vi "SIR2.vi"() -> ()   [LabVIEW 2014]
uses:
  <vilib>/Utility/file.llb/Write To Spreadsheet File (DBL).vi
  <vilib>/measure/mamon.llb/Waveform Peak Detection for 1 Chan.vi
  <vilib>/Utility/file.llb/Write To Spreadsheet File (string).vi
  <vilib>/Utility/file.llb/Read From Spreadsheet File (DBL).vi
  <vilib>/measure/NI_MAPro.lvlib
  <vilib>/Utility/file.llb/Read From Spreadsheet File (string).vi
panel:
  out "Feature ampltuides":dbl[][](array[numeric])
  out "Feature positions":dbl[][](array[numeric])
  out "teh data":refnum<data-value>
  out "Wavelengths":dbl[](array[numeric])
  in  "Load data":bool
  out "peaks/valleys":u16(ring) items=["Peaks", "Valleys"]
  out "Zero Ydata":sgl[](array[numeric])
  out "Zero Xdata":sgl[](array[numeric])
  out "ProgBar top":u32(slide) scale=-1.0..3016.0
  out "ProgBar bottom":u8(slide) scale=0.0..100.0
  in  "Run detection":bool
  in  "Delim":string
  out "Files":path[](array[path])
  in  "Ycol":i16=1
  in  "Xcol":i16
  in  "File style":u16(ring) items=["Sequential files", "Single database"]
  in  "Graph tab":T1(tab)
  out "Single scan":cluster{dbl[], dbl[]}[](graph)
  out "File\nname":string
  in  "Save single scan":bool
  in  "File displayed":i32(slide) min=0 max=5 step=1 scale=0.0..5.0
  in  "Save filtered spectras":bool
  out "Intensity Graph":dbl[][](graph)
  in  "Save Intensity plot":bool
  in  "Colour":string(combo)="Hot metal"
  out "Fixed point":cluster{i32[], dbl[]}(graph)
  in  "Save fixed point\ntracking":bool
  in  "Wavelength\nto track":dbl
  out "Closest wavelength":dbl
  out "Wavelength graph":dbl[][](graph)
  in  "Save Features":bool
  out "Intensity graph":dbl[][](graph)
  in  "Feature & tracking tabs":enum32{"Feature detection", "Tracking"}(tab)
  in  "Upper\nThreashold":dbl=20000.0
  in  "Lower\nThreashold":dbl
  in  "Width":dbl=20.0
  in  "2nd Derivative limit":dbl=0.01
  in  "Feature\ntype":string(combo)="1"
  in  "Detection method":string(combo)="0"
  in  "Feature\ndetection":bool
  in  "Open feature settings":bool
  in  "Tracking error limit":dbl=5.0 caption="Tracking error limit (%)"
  in  "Minimum feature length":i32=1
  in  "Tracking":bool
  in  "Tracking\ntype":string(combo)
  in  "Open Button 2":bool
  in  "Crop":bool
  in  "Normalise\nmethod":string(combo)
  in  "Normalise":bool
  in  "Decimate":i32
  in  "Decimate Y/N":bool
  in  "End\nwavelength":sgl
  in  "Start \nwavelength":sgl
  in  "Moving AV":bool
  in  "Transmission":bool
  in  "Load zero":bool
  in  "Moving\naverage":i16=1 min=1 step=1
  out "Number of files":i16
  in  "Load files":bool
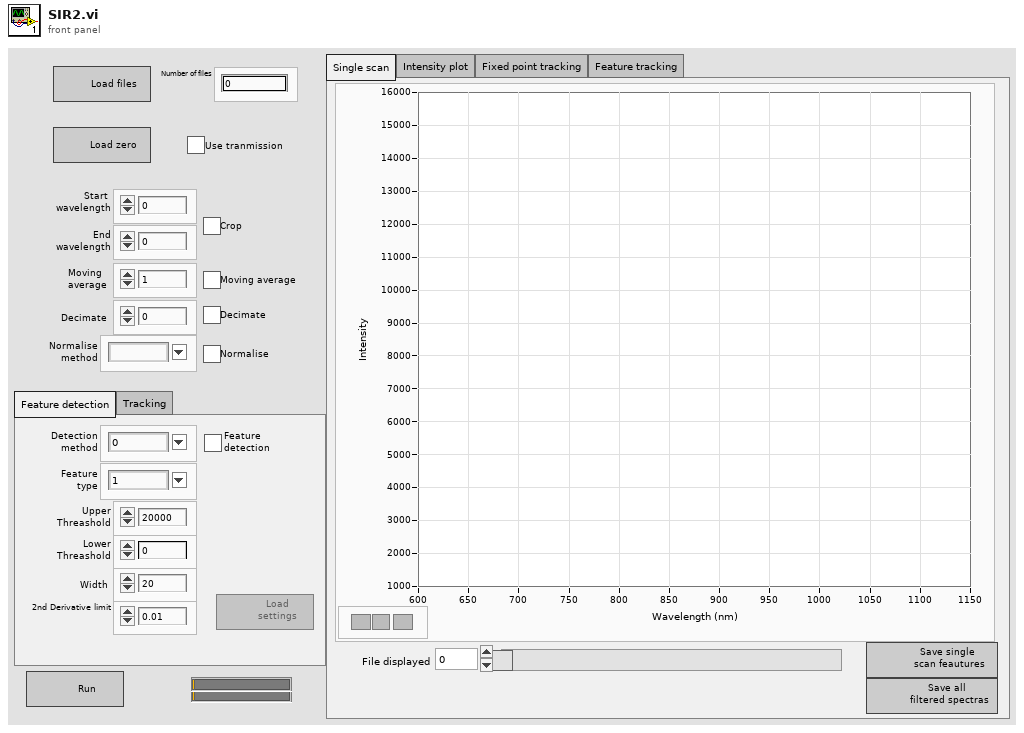
[diagram p1: front panel]
types:
  T1 = enum32{"Single scan", "Intensity plot", "Fixed point tracking", "Feature tracking"}
  T2 = cluster{"Feature positions":dbl[], "Feature ampltuides":dbl[]}
  T3 = cluster{"Feature positions":dbl[], "Feature ampltuides":dbl[]}[]
  T4 = typedef "imagedata.ctl" = cluster{"image type":i32, "image depth":i32, "image":u8[], "mask":u8[], "colors":u32[], "Rectangle":cluster{"left":i16, "top":i16, "right":i16, "bottom":i16}}
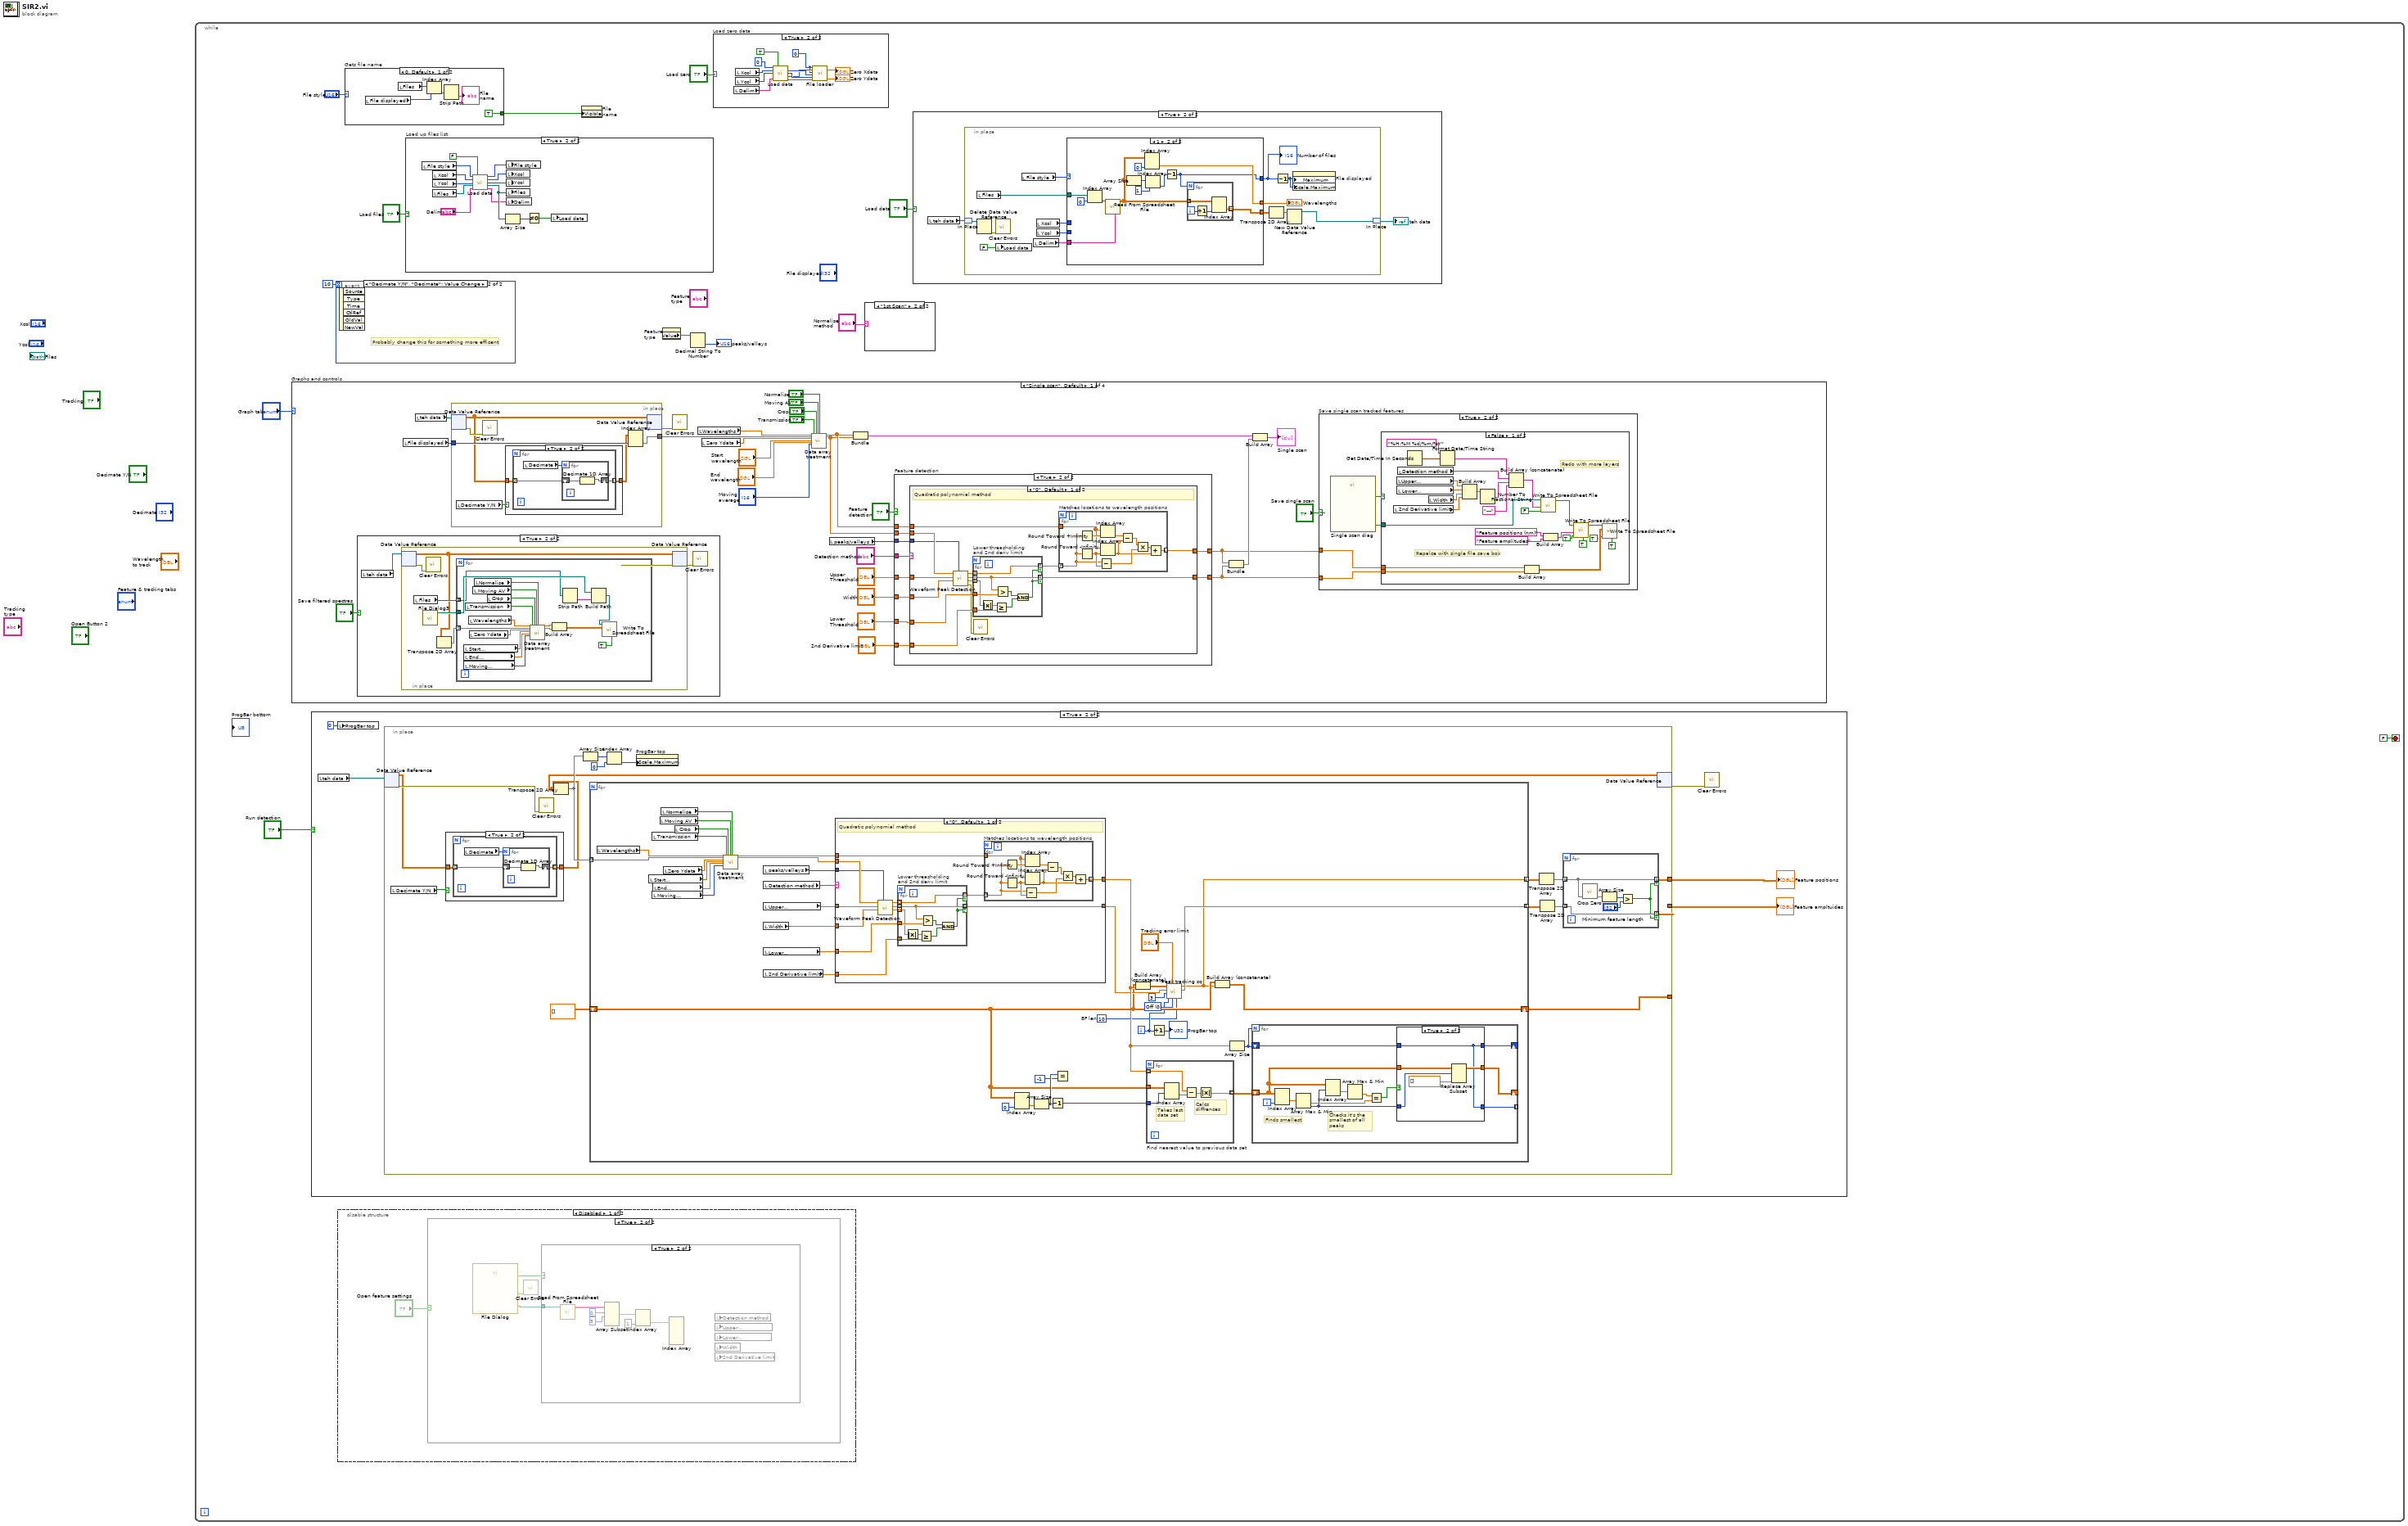
[diagram p0: block diagram]
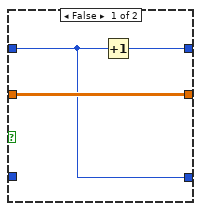
[diagram p7: hidden frame]
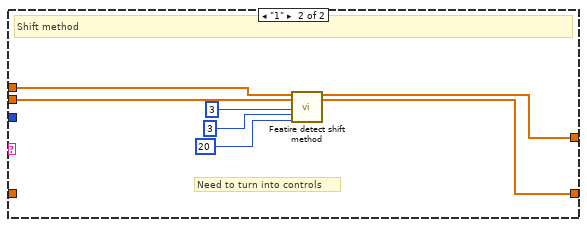
[diagram p8: hidden frame]
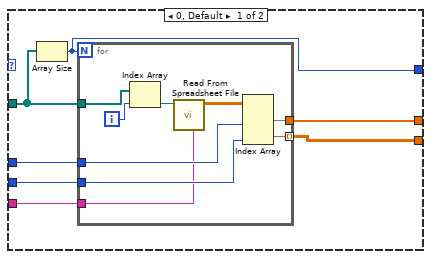
[diagram p10: hidden frame]
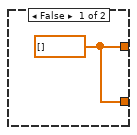
[diagram p17: hidden frame]
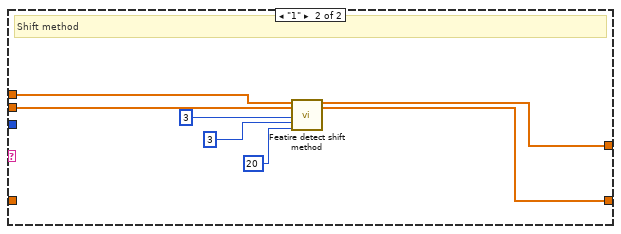
[diagram p18: hidden frame]
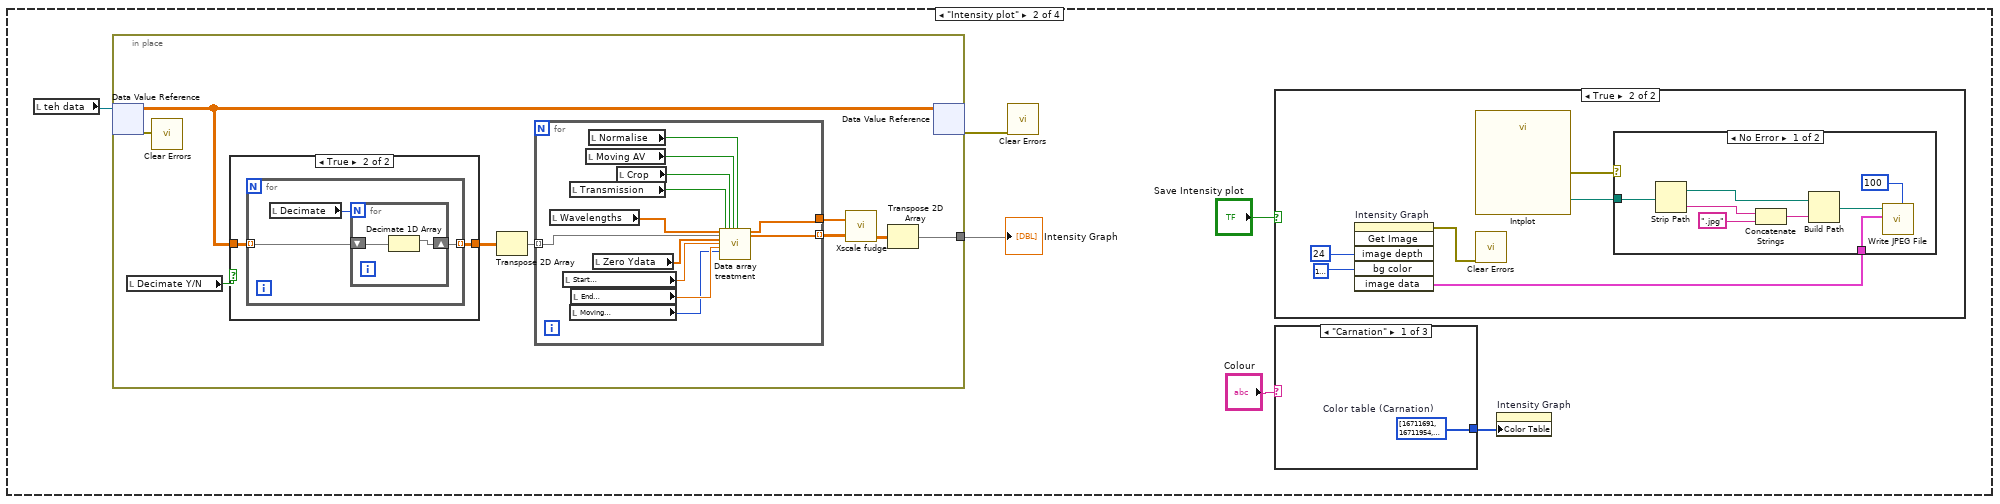
[diagram p19: hidden frame]
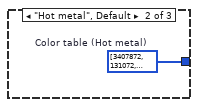
[diagram p20: hidden frame]
diagram:
  n1 = while {
    stop <- FALSE stop-if-true
    n2 = case "Graphs and controls" shown="\"Single scan\", Default" "Graph tab" {
      frame "Single scan", Default {
        n3 = case shown="True" "Save filtered spectras" {
          frame False {
          }
          frame True {
            n4 = local read "teh data"() -> (w252:refnum<data-value>)
            n5 = in-place {
              n6 = in-place-dvr #1(w252) -> (w254:dbl[][], w257:errorcluster)
              n7 = local read "Files"() -> (w256:path[])
              n8 = call "File Dialog3"() -> ("selected path"=w255:path)  [unwired: 12 in, 3 out]
              n9 = call <vilib>:"Clear Errors.vi"("error in (no error)"=w257) -> ()  [unwired: 5 in, 2 out]
              n10 = Transpose 2D Array(2D array=w254) -> (transposed array=w253:dbl[][])
              n11 = for {
                tunnel: w253 -> [w258] mode=indexing
                tunnel: w256 -> [w260] mode=indexing
                tunnel: w255 -> [w261]
                n12 = local read "Start \nwavelength"() -> (w273:sgl)
                n13 = local read "End\nwavelength"() -> (w272:sgl)
                n14 = local read "Moving\naverage"() -> (w271:i16)
                n15 = local read "Transmission"() -> (w270:bool)
                n16 = local read "Wavelengths"() -> (w275:dbl[])
                n17 = local read "Zero Ydata"() -> (w274:sgl[])
                n18 = local read "Moving AV"() -> (w268:bool)
                n19 = local read "Normalise"() -> (w267:bool)
                n20 = local read "Crop"() -> (w269:bool)
                n21 = call "Data array treatment.vi"("Xdata"=w275, "Ydata"=w258, "Zero array"=w274, "Start \nwavelength"=w273, "End\nwavelength"=w272, "Moving\naverage"=w271, "Transmission"=w270, "Crop"=w269, "Moving AV"=w268, "Normalise"=w267) -> ("Xdata"=w266:dbl[], "Ydata"=w265:dbl[])  [unwired: 16 in]
                n22 = Build Array(w266, w265) -> (w264:dbl[][])
                n23 = Strip Path(path=w260) -> (name=w262:string)  [unwired: 1 out]
                n24 = Build Path(base path=w261, name or relative path=w262) -> (appended path=w259:path)
                n25 = call-poly <vilib>:"Write To Spreadsheet File.vi"("transpose? (no:F)"=TRUE, "2D data"=w264, "file path (dialog if empty)"=w259) -> ()  [unwired: 5 in, 1 out]
              }
              n26 = in-place-dvr #1(w254) -> (w251:errorcluster)  [unwired: 1 out]
            }
            n27 = call <vilib>:"Clear Errors.vi"("error in (no error)"=w251) -> ()  [unwired: 5 in, 2 out]
          }
        }
        n28 = local read "File displayed"() -> (w228:i32)
        n29 = local read "teh data"() -> (w230:refnum<data-value>)
        n30 = in-place {
          in-place-border: w228 -> [w309]
          in-place-border: [w310] -> w226
          n31 = in-place-dvr #2(w230) -> (w308:dbl[][], w311:errorcluster)
          n32 = local read "Decimate Y/N"() -> (w306:bool)
          n33 = call <vilib>:"Clear Errors.vi"("error in (no error)"=w311) -> ()  [unwired: 5 in, 2 out]
          n34 = case shown="True" w306 {
            tunnel: w308 -> [w312 w314]
            tunnel: [w312 w313] -> w307
            frame False {
            }
            frame True {
              n35 = for {
                tunnel: [w316] -> w313 mode=indexing
                tunnel: w314 -> [w315] mode=indexing
                n36 = local read "Decimate"() -> (w317:i32)
                n37 = for {
                  N: w317 -> [_]
                  shift-right: [w318] -> w316
                  shift-left: w315 -> [w319]
                  n38 = Decimate 1D Array(w319) -> (w318:dbl[])  [unwired: 1 out]
                }
              }
            }
          }
          n39 = Index Array(array=w307, index (col)=w309) -> (element=w310:dbl[])  [unwired: 1 in]
          n40 = in-place-dvr #2(w308) -> (w229:errorcluster)  [unwired: 1 out]
        }
        n41 = call <vilib>:"Clear Errors.vi"("error in (no error)"=w229) -> ()  [unwired: 5 in, 2 out]
        n42 = local read "Wavelengths"() -> (w227:dbl[])
        n43 = local read "Zero Ydata"() -> (w231:sgl[])
        n44 = call "Data array treatment.vi"("Xdata"=w227, "Ydata"=w226, "Zero array"=w231, "Start \nwavelength"="Start \nwavelength", "End\nwavelength"="End\nwavelength", "Moving\naverage"="Moving\naverage", "Transmission"="Transmission", "Crop"="Crop", "Moving AV"="Moving AV", "Normalise"="Normalise") -> ("Xdata"=w240:dbl[], "Ydata"=w239:dbl[])  [unwired: 16 in]
        n45 = local read "peaks/valleys"() -> (w248:u16)
        n46 = Bundle("Xdata"=w240, "Ydata"=w239) -> (w241:cluster{"Xdata":dbl[], "Ydata":dbl[]})  [unwired: 1 in]
        n47 = case "Feature detection" shown="True" "Feature\ndetection" {
          tunnel: w240 -> [_ w329]
          tunnel: w239 -> [_ w328]
          tunnel: "Detection method" -> [_ w330]
          tunnel: w248 -> [_ w327]
          tunnel: "Upper\nThreashold" -> [_ w326]
          tunnel: "Width" -> [_ w325]
          tunnel: "Lower\nThreashold" -> [_ w324]
          tunnel: "2nd Derivative limit" -> [_ w323]
          tunnel: [w320 w322] -> w224
          tunnel: [w320 w321] -> w223
          frame False {
            w320 = dbl[] []
          }
          frame True {
            n48 = case shown="\"0\", Default" w330 {
              tunnel: w329 -> [w334 w370]
              tunnel: w328 -> [w344 w369]
              tunnel: w327 -> [w343 _]
              tunnel: w326 -> [w342 _]
              tunnel: w325 -> [w341 _]
              tunnel: w324 -> [w337 _]
              tunnel: w323 -> [w336 _]
              tunnel: [w333 w368] -> w321
              tunnel: [w332 w367] -> w322
              frame "0", Default {
                # "Quadratic polynomial method"
                n49 = call-poly <vilib>:"Waveform Peak Detection.vi"("peaks/valleys"=w343, "width"=w341, "threshold"=w342, "Signal In"=w344) -> ("error out"=w331:errorcluster, "2nd Derivatives"=w338:dbl[], "Amplitudes"=w339:dbl[], "Locations"=w340:dbl[])  [unwired: 3 in, 1 out]
                n50 = for "Lower threasholding\nand 2nd deriv limit" {
                  tunnel: w340 -> [w362] mode=indexing
                  tunnel: w339 -> [w361] mode=indexing
                  tunnel: w338 -> [w355] mode=indexing
                  tunnel: w337 -> [w363]
                  tunnel: [w362] -> w335 mode=indexing if=w360
                  tunnel: [w361] -> w332 mode=indexing if=w360
                  tunnel: w336 -> [w359]
                  n51 = Absolute Value(x=w355) -> (abs(x)=w356:dbl)
                  n52 = Greater Or Equal?(x=w356, y=w359) -> (x >= y?=w358:bool)
                  n53 = Greater?(x=w361, y=w363) -> (0:w357:bool)
                  n54 = And(x=w357, y=w358) -> (x .and. y?=w360:bool)
                }
                n55 = call <vilib>:"Clear Errors.vi"("error in (no error)"=w331) -> ()  [unwired: 5 in, 2 out]
                n56 = for "Matches locations to wavelength positions" {
                  tunnel: w335 -> [w346] mode=indexing
                  tunnel: w334 -> [w347]
                  tunnel: [w345] -> w333 mode=indexing
                  n57 = Round Toward +Infinity ("Round To +Infinity")(x=w346) -> (ceil(x): smallest int >= x=w354:dbl)
                  n58 = Round Toward -Infinity ("Round To -Infinity")(1:w346) -> (0:w353:dbl)
                  n59 = Subtract(x=w346, y=w353) -> (x-y=w350:dbl)
                  n60 = Index Array(array=w347, index=w354) -> (element=w352:dbl)
                  n61 = Index Array(array=w347, index=w353) -> (element=w348:dbl)
                  n62 = Subtract(x=w352, y=w348) -> (x-y=w351:dbl)
                  n63 = Multiply(x=w351, y=w350) -> (x*y=w349:dbl)
                  n64 = Add(x=w349, y=w348) -> (x+y=w345:dbl)
                }
              }
              frame "1" {
                # "Shift method"
                n65 = call "Featire detect shift method.vi"("Xvalues"=w370, "Yvalues"=w369, "magnitude  limit"=3, "Shift"=3, "Window"=20) -> ("Feature positions"=w368:dbl[], "Feature ampltuides"=w367:dbl[])  [unwired: 13 in]
              }
            }
          }
        }
        n66 = Bundle("Feature positions"=w223, "Feature ampltuides"=w224) -> (w242:T2)  [unwired: 1 in]
        n67 = Build Array(w241, w242) -> (→"Single scan":T3)
        n68 = case "Save single scan tracked features" shown="True" "Save single scan" {
          tunnel: w224 -> [_ w277]
          tunnel: w223 -> [_ w276]
          frame False {
          }
          frame True {
            n69 = call "Single scan diag"() -> ("selected path"=w279:path, "cancelled"=w278:bool)  [unwired: 12 in, 2 out]
            n70 = case shown="False" w278 {
              tunnel: w279 -> [w287 _]
              tunnel: w277 -> [w296 _]
              tunnel: w276 -> [w295 _]
              frame False {
                # "Repalce with single file save box"
                # "Redo with more layers"
                n71 = local read "2nd Derivative limit"() -> (w291:dbl)
                n72 = local read "Upper\nThreashold"() -> (w288:dbl)
                n73 = local read "Lower\nThreashold"() -> (w289:dbl)
                n74 = local read "Detection method"() -> (w293:string)
                n75 = Get Date/Time In Seconds() -> (seconds since 1Jan1904=w282:timestamp)
                n76 = local read "Width"() -> (w290:dbl)
                n77 = Format Date/Time String(time format string (%c)="%H:%M %d/%m/%Y", seconds (now)=w282) -> (date/time string=w283:string)  [unwired: 1 in]
                n78 = Build Array(w288, w289, w290, w291) -> (w292:dbl[])
                n79 = Number To Fractional String(number=w292) -> (F-format string=w294:string[])  [unwired: 3 in]
                n80 = Build Array (concatenate)(w283, w293, w294, "---") -> (w285:string[])
                n81 = Build Array(w295, w296) -> (w300:dbl[][])
                n82 = call-poly <vilib>:"Write To Spreadsheet File.vi"("append to file? (new file:F)"=FALSE, "1D data"=w285, "file path (dialog if empty)"=w287) -> ("new file path (Not A Path if cancelled)"=w286:path)  [unwired: 5 in]
                n83 = Build Array("Feature positions (nm)", "Feature amplitudes") -> (w299:string[])
                n84 = call-poly <vilib>:"Write To Spreadsheet File.vi"("transpose? (no:F)"=TRUE, "append to file? (new file:F)"=TRUE, "1D data"=w299, "file path (dialog if empty)"=w286) -> ("new file path (Not A Path if cancelled)"=w305:path)  [unwired: 4 in]
                n85 = call-poly <vilib>:"Write To Spreadsheet File.vi"("transpose? (no:F)"=TRUE, "append to file? (new file:F)"=TRUE, "2D data"=w300, "file path (dialog if empty)"=w305) -> ()  [unwired: 4 in, 1 out]
              }
              frame True {
              }
            }
          }
        }
      }
      frame "Intensity plot" {
        n86 = local read "teh data"() -> (w376:refnum<data-value>)
        n87 = in-place {
          in-place-border: [w399] -> w374
          n88 = in-place-dvr #3(w376) -> (w394:dbl[][], w398:errorcluster)
          n89 = local read "Decimate Y/N"() -> (w396:bool)
          n90 = call <vilib>:"Clear Errors.vi"("error in (no error)"=w398) -> ()  [unwired: 5 in, 2 out]
          n91 = case shown="True" w396 {
            tunnel: [w403 w405] -> w395
            tunnel: w394 -> [w403 w404]
            frame False {
            }
            frame True {
              n92 = for {
                tunnel: [w407] -> w405 mode=indexing
                tunnel: w404 -> [w406] mode=indexing
                n93 = local read "Decimate"() -> (w408:i32)
                n94 = for {
                  N: w408 -> [_]
                  shift-right: [w409] -> w407
                  shift-left: w406 -> [w410]
                  n95 = Decimate 1D Array(w410) -> (w409:dbl[])  [unwired: 1 out]
                }
              }
            }
          }
          n96 = Transpose 2D Array(2D array=w395) -> (transposed array=w397:dbl[][])
          n97 = for {
            tunnel: [w414] -> w402 mode=indexing
            tunnel: [w413] -> w401
            tunnel: w397 -> [w412] mode=indexing
            n98 = local read "Wavelengths"() -> (w411:dbl[])
            n99 = local read "Start \nwavelength"() -> (w418:sgl)
            n100 = local read "Transmission"() -> (w419:bool)
            n101 = local read "Moving\naverage"() -> (w416:i16)
            n102 = local read "End\nwavelength"() -> (w417:sgl)
            n103 = local read "Moving AV"() -> (w421:bool)
            n104 = local read "Normalise"() -> (w422:bool)
            n105 = local read "Zero Ydata"() -> (w415:sgl[])
            n106 = local read "Crop"() -> (w420:bool)
            n107 = call "Data array treatment.vi"("Xdata"=w411, "Ydata"=w412, "Zero array"=w415, "Start \nwavelength"=w418, "End\nwavelength"=w417, "Moving\naverage"=w416, "Transmission"=w419, "Crop"=w420, "Moving AV"=w421, "Normalise"=w422) -> ("Xdata"=w413:dbl[], "Ydata"=w414:dbl[])  [unwired: 16 in]
          }
          n108 = call "Xscale fudge.vi"("x array"=w401, "intensity array in"=w402) -> ("intensity array out"=w400:dbl[][])  [unwired: 2 out]
          n109 = Transpose 2D Array(2D array=w400) -> (transposed array=w399:dbl[][])
          n110 = in-place-dvr #3(w394) -> (w375:errorcluster)  [unwired: 1 out]
        }
        "Intensity Graph" <- w374
        n111 = call <vilib>:"Clear Errors.vi"("error in (no error)"=w375) -> ()  [unwired: 5 in, 2 out]
        n112 = case shown="True" "Save Intensity plot" {
          frame False {
          }
          frame True {
            n113 = invoke on="Intensity Graph" class="IntGraph (strict)" method="Get Image"("image depth"=24 ("Image Depth"), "bg color"=u32 16777225) -> (error out=w383:errorcluster, "image data"=w382:T4)  [unwired: 4 in, 4 out]
            n114 = call "Intplot"() -> ("selected path"=w381:path, "error out"=w384:errorcluster)  [unwired: 12 in, 2 out]
            n115 = call <vilib>:"Clear Errors.vi"("error in (no error)"=w383) -> ()  [unwired: 5 in, 2 out]
            n116 = case shown="No Error" w384 {
              tunnel: w381 -> [w392 _]
              tunnel: w382 -> [w386 _]
              frame No Error {
                n117 = Strip Path(path=w392) -> (stripped path=w388:path, name=w390:string)
                n118 = Concatenate Strings(w390, ".jpg") -> (w389:string)
                n119 = Build Path(base path=w388, name or relative path=w389) -> (appended path=w387:path)
                n120 = call <vilib>:"Write JPEG File.vi"("quality (80)"=100, "image data"=w386, "path to JPEG file"=w387) -> ()  [unwired: 7 in, 2 out]
              }
              frame Error {
              }
            }
          }
        }
        n121 = case shown="\"Carnation\"" "Colour" {
          tunnel: [w377 w378 w379] -> w371
          frame "Carnation" {
            w377 = u32[] [16711691, 16711954, 16712217, 16712480, 16712742, 16713005, 16713268, 16713530, 16713793, 16714056, 16715086, 16714580, 16714842, 16715104, 16715367, 16715629, 16715891, 16716153, 16716415, 16716677, 16716940, 16717202, 16717463, 16717725, 16717987, 16718249, 16718511, 16718772, 16719034, 16719296, 16719557, 16719819, 16720079, 16720341, 16720602, 16720863, 16721125, 16721386, 16721647, 16721908, 16722169, 16722430, 16395007, 16133119, 15805695, 15478271, 15216383, 14888959, 14561535, 14234111, 13972223, 13644799, 13382911, 13055487, 12793599, 12531711, 12269823, 11942399, 11680511, 11418623, 11156735, 10829311, 10567423, 10305535, 10305535, 10043647, 9781503, 9585151, 9323263, 9061375, 8799487, 8537599, 8341247, 8079359, 7883007, 7621119, 7424767, 7228415, 6966527, 6770175, 6573823, 6377471, 6115583, 5919231, 5722879, 5526527, 5527551, 5594111, 5660927, 5727743, 5794559, 5861375, 5927935, 5994751, 6061567, 6128127, 6194943, 6261503, 6328063, 6394879, 6461439, 6527999, 6594815, 6661375, 6727935, 6794495, 6861055, 6927871, 6994175, 7060735, 7127295, 7193855, 7260415, 7326719, 7393279, 7459839, 7526143, 7592703, 7659007, 7725311, 7791871, 7858175, 7924479, 7991039, 8057343, 8123647, 8189951, 8256255, 8322815, 8388605, 8454139, 8519672, 8585205, 8650738, 8716271, 8781804, 8847338, 8912871, 8978404, 9043938, 9109472, 9175005, 9240539, 9306073, 9371606, 9437140, 9502674, 9568208, 9633742, 9699275, 9764809, 9830343, 9895877, 9961412, 10026946, 10092480, 10158014, 10223548, 10289083, 10354617, 10420152, 10485686, 10551221, 10616755, 10682290, 10747825, 10813359, 10878894, 10944429, 11009964, 11075499, 11141034, 11206570, 11403179, 11599788, 11796397, 11993006, 12124079, 12320688, 12517297, 12648370, 12844979, 13041588, 13172661, 13303734, 13500343, 13631416, 13762489, 13959098, 14090171, 14221244, 14352317, 14352317, 14483390, 14614463, 14745535, 14876608, 15007681, 15138754, 15269827, 15335364, 15466437, 15597510, 15663047, 15794120, 15859657, 15990730, 16056267, 16121804, 16252877, 16318414, 16383951, 16515024, 16580561, 16646098, 16711635, 16776916, 16776917, 16776662, 16776407, 16776152, 16775897, 16775642, 16775643, 16775388, 16775133, 16775134, 16775135, 16774880, 16774881, 16774626, 16774627, 16774628, 16774373, 16774374, 16774375, 16774376, 16774377, 16774378, 16774379, 16774380, 16774381, 16774638, 16774639, 16774640, 16774641, 16774898, 16774899, 16775156, 16775157, 16775414, 16775415, 16775672, 16775929, 16776186, 16776187]  # Color table (Carnation)
          }
          frame "Hot metal", Default {
            w378 = u32[] [3407872, 131072, 196608, 327680, 458752, 589824, 655360, 786432, 917504, 1048576, 1114112, 1245184, 1376256, 1507328, 1572864, 1703936, 1835008, 1966080, 2031616, 2162688, 2293760, 2424832, 2555904, 2621440, 2752512, 2883584, 3014656, 3080192, 3211264, 3342336, 3473408, 3538944, 3670016, 3801088, 3932160, 3997696, 4128768, 4259840, 4390912, 4456448, 4587520, 4718592, 4849664, 4980736, 5046272, 5177344, 5308416, 5439488, 5505024, 5636096, 5767168, 5898240, 5963776, 6094848, 6225920, 6356992, 6422528, 6553600, 6684672, 6815744, 6881280, 7012352, 7143424, 7143424, 7274496, 7405568, 7471104, 7602176, 7733248, 7864320, 7929856, 8060928, 8192000, 8323072, 8388608, 8519680, 8650752, 8781824, 8847360, 8978432, 9109504, 9240576, 9306112, 9437184, 9568256, 9699328, 9830400, 9895936, 10027008, 10158080, 10289152, 10354688, 10485760, 10616832, 10747904, 10813440, 10944512, 11075584, 11206656, 11272192, 11403264, 11534336, 11665408, 11730944, 11862016, 11993088, 12124160, 12189696, 12320768, 12451840, 12582912, 12713984, 12779520, 12910592, 13041664, 13172736, 13238272, 13369344, 13500416, 13631488, 13697024, 13828096, 13959168, 14090240, 14155776, 14286848, 14417920, 14548992, 14614528, 14745600, 14876672, 15007744, 15138816, 15204352, 15335424, 15466496, 15597568, 15663104, 15794176, 15925248, 16056320, 16121856, 16252928, 16384000, 16515072, 16580608, 16580608, 16580608, 16515072, 16711680, 16711680, 16711680, 16712192, 16647424, 16713728, 16714496, 16715264, 16716032, 16716800, 16717568, 16718336, 16719104, 16719872, 16720640, 16721408, 16722176, 16722944, 16723712, 16724480, 16725248, 16726016, 16726784, 16727552, 16728064, 16728832, 16729600, 16730368, 16731136, 16731904, 16732672, 16733440, 16734208, 16734976, 16735744, 16736512, 16737280, 16738048, 16738816, 16739584, 16740352, 16741120, 16741120, 16741888, 16742656, 16743424, 16743936, 16744704, 16745472, 16746240, 16747008, 16747776, 16748544, 16749312, 16750080, 16750848, 16751616, 16752384, 16753152, 16753920, 16754688, 16755456, 16756224, 16756992, 16757760, 16758528, 16759296, 16760064, 16760576, 16761344, 16762112, 16762880, 16763648, 16764416, 16765184, 16765952, 16766720, 16767488, 16768256, 16769024, 16769792, 16770560, 16771328, 16772096, 16772864, 16773632, 16774400, 16775168, 16775936, 16776448, 16776960, 16776960, 16776960, 16776960, 16776960, 16776960, 16776960, 16776960, 16776960, 16776960, 16776960, 16776960, 16776960, 16776960, 16776960, 16776448]  # Color table (Hot metal)
          }
          frame "Rainbow-striped" {
            w379 = u32[] [12255418, 12386492, 12517567, 12320960, 12189888, 12058817, 11927746, 11731139, 11600067, 9175197, 9044125, 11141318, 11010246, 10813639, 10682568, 10551497, 10354890, 10223818, 10092747, 7930019, 7798948, 9633997, 9502926, 9306319, 9175248, 9044176, 8847569, 8716498, 8585427, 6750377, 6619306, 8126677, 7995606, 7798999, 7667927, 7536856, 7340249, 7209178, 7078106, 5505199, 5374128, 6619357, 6488285, 6291678, 6160607, 6029536, 5832929, 5701857, 5570786, 4325557, 4194486, 5112036, 4980965, 4784358, 4653287, 4522215, 4325608, 4194537, 4063466, 3080380, 3014844, 3604716, 3408109, 3277038, 3277038, 3145966, 3014895, 2818288, 2687217, 2556145, 1900738, 1769666, 2097396, 1900789, 1769717, 1638646, 1507575, 1310968, 1179896, 1048825, 721096, 590024, 590075, 393468, 262397, 131326, 255, 1791, 3327, 4863, 5068, 6348, 9471, 11007, 12543, 14079, 15615, 17151, 18687, 20223, 17612, 18636, 25087, 26623, 28159, 29695, 31231, 32767, 34303, 35839, 29900, 31180, 40447, 41983, 43775, 45311, 46847, 48383, 49919, 51455, 42444, 43724, 56063, 57599, 59135, 60671, 62207, 63743, 65535, 65528, 52418, 52413, 65510, 65504, 65498, 65492, 65486, 65480, 65474, 65468, 52369, 52364, 65449, 65443, 65437, 65431, 65425, 65419, 65413, 65407, 52321, 52316, 65389, 65383, 65377, 65371, 65364, 65358, 65352, 65346, 52272, 52267, 65328, 65322, 65316, 65310, 65304, 65298, 65292, 65286, 52224, 314368, 851712, 1244928, 1638144, 2031360, 2424576, 2817792, 3211008, 3604224, 3197952, 3525632, 4783872, 5177088, 5635840, 6029056, 6422272, 6815488, 7208704, 7601920, 6409216, 6736896, 6736896, 8781568, 9174784, 9568000, 9961216, 10354432, 10747648, 11206400, 11599616, 9554944, 9882624, 12779264, 13172480, 13565696, 13958912, 14352128, 14745344, 15138560, 15531776, 12766208, 13093888, 16776960, 16775170, 16773637, 16771847, 16770314, 16768780, 16766991, 16765457, 13411088, 13409810, 16760601, 16758812, 16757278, 16755745, 16753955, 16752422, 16750888, 16749099, 13398052, 13396774, 16744243, 16742704, 16741166, 16739884, 16738345, 16736807, 16735269, 16733730, 13385753, 13384728, 16729371, 16727833, 16726295, 16725012, 16723474, 16721936, 16720397, 16718859, 13373959, 13372677, 16714500, 16712962, 16711680]  # Color table (Rainbow-striped)
          }
        }
        n122 = property on="Intensity Graph" class="IntGraph (strict)"("Color Table"=w371) -> ()  [unwired: 2 in, 2 out]
      }
      frame "Fixed point tracking" {
        n123 = local read "teh data"() -> (w427:refnum<data-value>)
        n124 = in-place {
          in-place-border: [w453] -> w428
          in-place-border: [w446] -> w425
          in-place-border: [w445] -> w423
          n125 = in-place-dvr #4(w427) -> (w448:dbl[][], w451:errorcluster)
          n126 = local read "Decimate Y/N"() -> (w447:bool)
          n127 = call <vilib>:"Clear Errors.vi"("error in (no error)"=w451) -> ()  [unwired: 5 in, 2 out]
          n128 = case shown="True" w447 {
            tunnel: [w455 w457] -> w449
            tunnel: w448 -> [w455 w456]
            frame False {
            }
            frame True {
              n129 = for {
                tunnel: [w459] -> w457 mode=indexing
                tunnel: w456 -> [w458] mode=indexing
                n130 = local read "Decimate"() -> (w460:i32)
                n131 = for {
                  N: w460 -> [_]
                  shift-right: [w461] -> w459
                  shift-left: w458 -> [w462]
                  n132 = Decimate 1D Array(w462) -> (w461:dbl[])  [unwired: 1 out]
                }
              }
            }
          }
          n133 = local read "Wavelengths"() -> (w452:dbl[])
          n134 = Transpose 2D Array(2D array=w449) -> (transposed array=w450:dbl[][])
          n135 = local read "Wavelength\nto track"() -> (w454:dbl)
          n136 = for {
            tunnel: w454 -> [w471]
            tunnel: [w467] -> w445 mode=indexing
            tunnel: [w466] -> w446 mode=indexing
            tunnel: w452 -> [w465]
            tunnel: w450 -> [w464] mode=indexing
            i -> [w466]
            n137 = local read "Start \nwavelength"() -> (w475:sgl)
            n138 = local read "Moving\naverage"() -> (w473:i16)
            n139 = local read "End\nwavelength"() -> (w474:sgl)
            n140 = local read "Transmission"() -> (w476:bool)
            n141 = local read "Zero Ydata"() -> (w472:sgl[])
            n142 = local read "Moving AV"() -> (w478:bool)
            n143 = local read "Normalise"() -> (w479:bool)
            n144 = local read "Crop"() -> (w477:bool)
            n145 = call "Data array treatment.vi"("Xdata"=w465, "Ydata"=w464, "Zero array"=w472, "Start \nwavelength"=w475, "End\nwavelength"=w474, "Moving\naverage"=w473, "Transmission"=w476, "Crop"=w477, "Moving AV"=w478, "Normalise"=w479) -> ("Xdata"=w470:dbl[], "Ydata"=w469:dbl[])  [unwired: 16 in]
            n146 = call "Search 1D Array for Nearest.vi"("desired element"=w471, "1D Array"=w470) -> ("closest index"=w468:i32, "closest element"=→"Closest wavelength":dbl)  [unwired: 8 in]
            n147 = Index Array(array=w469, index=w468) -> (element=w467:dbl)
          }
          n148 = Bundle(w446, w445) -> (w453:cluster{i32[], dbl[]})  [unwired: 1 in]
          n149 = in-place-dvr #4(w448) -> (w426:errorcluster)  [unwired: 1 out]
        }
        "Fixed point" <- w428
        n150 = call <vilib>:"Clear Errors.vi"("error in (no error)"=w426) -> ()  [unwired: 5 in, 2 out]
        n151 = case shown="True" "Save fixed point\ntracking" {
          tunnel: w425 -> [_ w430]
          tunnel: w423 -> [_ w429]
          frame False {
          }
          frame True {
            n152 = call "Fixed point diag"() -> ("selected path"=w432:path, "cancelled"=w431:bool)  [unwired: 12 in, 2 out]
            n153 = case shown="False" w431 {
              tunnel: w432 -> [w433 _]
              tunnel: w430 -> [w435 _]
              tunnel: w429 -> [w434 _]
              frame False {
                n154 = Build Array("File", "Amplitude") -> (w442:string[])
                n155 = Build Array(w435, w434) -> (w441:dbl[][])
                n156 = call-poly <vilib>:"Write To Spreadsheet File.vi"("transpose? (no:F)"=TRUE, "append to file? (new file:F)"=FALSE, "1D data"=w442, "file path (dialog if empty)"=w433) -> ("new file path (Not A Path if cancelled)"=w436:path)  [unwired: 4 in]
                n157 = call-poly <vilib>:"Write To Spreadsheet File.vi"("transpose? (no:F)"=TRUE, "append to file? (new file:F)"=TRUE, "2D data"=w441, "file path (dialog if empty)"=w436) -> ()  [unwired: 4 in, 1 out]
              }
              frame True {
              }
            }
          }
        }
      }
      frame "Feature tracking" {
        n158 = local read "Feature ampltuides"() -> (w482:dbl[][])
        "Intensity graph" <- w482
        n159 = local read "Feature positions"() -> (w481:dbl[][])
        "Wavelength graph" <- w481
        n160 = case shown="True" "Save Features" {
          tunnel: w482 -> [_ w489]
          tunnel: w481 -> [_ w490]
          frame False {
          }
          frame True {
            n161 = for {
              tunnel: w490 -> [w503] mode=indexing
              tunnel: w489 -> [w502] mode=indexing
              shift-right: [w501] -> w488
              shift-left: dbl[][] [] -> [w500]
              n162 = Build Array (concatenate)(w500, w503, w502) -> (w501:dbl[][])
            }
            n163 = Transpose 2D Array(2D array=w488) -> (transposed array=w484:dbl[][])
            n164 = call "File Dialog2"() -> ("selected path"=w485:path, "cancelled"=w487:bool, "error out"=w486:errorcluster)  [unwired: 12 in, 1 out]
            n165 = call <vilib>:"Clear Errors.vi"("error in (no error)"=w486) -> ()  [unwired: 5 in, 2 out]
            n166 = case shown="False" w487 {
              tunnel: w485 -> [w493 _]
              tunnel: w484 -> [w491 _]
              frame False {
                n167 = Get Date/Time In Seconds() -> (seconds since 1Jan1904=w496:timestamp)
                n168 = Format Date/Time String(time format string (%c)="%H:%M %d/%m/%Y", seconds (now)=w496) -> (date/time string=w495:string)  [unwired: 1 in]
                n169 = Build Array(w495) -> (w494:string[])
                n170 = call-poly <vilib>:"Write To Spreadsheet File.vi"("append to file? (new file:F)"=FALSE, "1D data"=w494, "file path (dialog if empty)"=w493) -> ("new file path (Not A Path if cancelled)"=w492:path)  [unwired: 5 in]
                n171 = call-poly <vilib>:"Write To Spreadsheet File.vi"("append to file? (new file:F)"=TRUE, "2D data"=w491, "file path (dialog if empty)"=w492) -> ()  [unwired: 5 in, 1 out]
              }
              frame True {
              }
            }
          }
        }
      }
    }
    n172 = case shown="True" "Run detection" {
      frame False {
      }
      frame True {
        n173 = local read "teh data"() -> (w28:refnum<data-value>)
        n174 = local write "ProgBar top"(0) -> ()
        n175 = in-place {
          in-place-border: [w37] -> w25
          in-place-border: [w36] -> w24
          in-place-border: [w42] -> _
          n176 = in-place-dvr #5(w28) -> (w30:dbl[][], w44:errorcluster)
          n177 = local read "Decimate Y/N"() -> (w31:bool)
          n178 = case shown="True" w31 {
            tunnel: w30 -> [w45 w47]
            tunnel: [w45 w46] -> w29
            frame False {
            }
            frame True {
              n179 = for {
                tunnel: [w49] -> w46 mode=indexing
                tunnel: w47 -> [w48] mode=indexing
                n180 = local read "Decimate"() -> (w50:i32)
                n181 = for {
                  N: w50 -> [_]
                  shift-right: [w51] -> w49
                  shift-left: w48 -> [w52]
                  n182 = Decimate 1D Array(w52) -> (w51:dbl[])  [unwired: 1 out]
                }
              }
            }
          }
          n183 = call <vilib>:"Clear Errors.vi"("error in (no error)"=w44) -> ()  [unwired: 5 in, 2 out]
          n184 = Transpose 2D Array(2D array=w29) -> (transposed array=w41:dbl[][])
          n185 = Array Size(array=w41) -> (size(s)=w40:i32[])
          n186 = for {
            tunnel: [w62] -> w35 mode=indexing
            tunnel: [w63] -> w33 mode=indexing
            tunnel: w41 -> [w79] mode=indexing
            shift-right: [w64] -> w42
            shift-left: dbl[][] [] ("Feature positions") -> [w65]
            i -> [w61]
            w59 = 10  # BF len
            w66 = u16 0 items=["Off", "Linear best fit", "Polynomial best fit", "Moving average"] ("EnH choice")
            n187 = local read "Wavelengths"() -> (w88:dbl[])
            n188 = local read "Start \nwavelength"() -> (w92:sgl)
            n189 = local read "Transmission"() -> (w93:bool)
            n190 = local read "Moving\naverage"() -> (w90:i16)
            n191 = local read "End\nwavelength"() -> (w91:sgl)
            n192 = local read "Moving AV"() -> (w95:bool)
            n193 = local read "Normalise"() -> (w96:bool)
            n194 = local read "Zero Ydata"() -> (w89:sgl[])
            n195 = local read "Crop"() -> (w94:bool)
            n196 = call "Data array treatment.vi"("Xdata"=w88, "Ydata"=w79, "Zero array"=w89, "Start \nwavelength"=w92, "End\nwavelength"=w91, "Moving\naverage"=w90, "Transmission"=w93, "Crop"=w94, "Moving AV"=w95, "Normalise"=w96) -> ("Xdata"=w81:dbl[], "Ydata"=w80:dbl[])  [unwired: 16 in]
            n197 = local read "peaks/valleys"() -> (w87:u16)
            n198 = local read "Detection method"() -> (w82:string)
            n199 = local read "Upper\nThreashold"() -> (w83:dbl)
            n200 = local read "Width"() -> (w84:dbl)
            n201 = local read "Lower\nThreashold"() -> (w85:dbl)
            n202 = local read "2nd Derivative limit"() -> (w86:dbl)
            n203 = case shown="\"0\", Default" w82 {
              tunnel: w81 -> [w125 w161]
              tunnel: w80 -> [w135 w160]
              tunnel: w87 -> [w134 _]
              tunnel: w83 -> [w133 _]
              tunnel: w84 -> [w132 _]
              tunnel: w85 -> [w128 _]
              tunnel: w86 -> [w127 _]
              tunnel: [w124 w159] -> w69
              tunnel: [w123 w158] -> w68
              frame "0", Default {
                # "Quadratic polynomial method"
                n204 = call-poly <vilib>:"Waveform Peak Detection.vi"("peaks/valleys"=w134, "width"=w132, "threshold"=w133, "Signal In"=w135) -> ("2nd Derivatives"=w129:dbl[], "Amplitudes"=w130:dbl[], "Locations"=w131:dbl[])  [unwired: 3 in, 2 out]
                n205 = for "Lower threasholding\nand 2nd deriv limit" {
                  tunnel: w131 -> [w153] mode=indexing
                  tunnel: w130 -> [w152] mode=indexing
                  tunnel: w129 -> [w146] mode=indexing
                  tunnel: w128 -> [w154]
                  tunnel: [w153] -> w126 mode=indexing if=w151
                  tunnel: [w152] -> w123 mode=indexing if=w151
                  tunnel: w127 -> [w150]
                  n206 = Absolute Value(x=w146) -> (abs(x)=w147:dbl)
                  n207 = Greater Or Equal?(x=w147, y=w150) -> (x >= y?=w149:bool)
                  n208 = Greater?(x=w152, y=w154) -> (0:w148:bool)
                  n209 = And(x=w148, y=w149) -> (x .and. y?=w151:bool)
                }
                n210 = for "Matches locations to wavelength positions" {
                  tunnel: w126 -> [w137] mode=indexing
                  tunnel: w125 -> [w138]
                  tunnel: [w136] -> w124 mode=indexing
                  n211 = Round Toward +Infinity ("Round To +Infinity")(x=w137) -> (ceil(x): smallest int >= x=w145:dbl)
                  n212 = Round Toward -Infinity ("Round To -Infinity")(1:w137) -> (0:w144:dbl)
                  n213 = Subtract(x=w137, y=w144) -> (x-y=w141:dbl)
                  n214 = Index Array(array=w138, index=w145) -> (element=w143:dbl)
                  n215 = Index Array(array=w138, index=w144) -> (element=w139:dbl)
                  n216 = Subtract(x=w143, y=w139) -> (x-y=w142:dbl)
                  n217 = Multiply(x=w142, y=w141) -> (x*y=w140:dbl)
                  n218 = Add(x=w140, y=w139) -> (x+y=w136:dbl)
                }
              }
              frame "1" {
                # "Need to turn into controls"
                # "Shift method"
                n219 = call "Featire detect shift method.vi"("Xvalues"=w161, "Yvalues"=w160, "magnitude  limit"=3, "Shift"=3, "Window"=20) -> ("Feature positions"=w159:dbl[], "Feature ampltuides"=w158:dbl[])  [unwired: 13 in]
              }
            }
            n220 = Index Array(array=w65, index (col)=0) -> (element=w76:dbl[])  [unwired: 1 in]
            n221 = Array Size(array=w76) -> (size(s)=w72:i32)
            n222 = Decrement(x=w72) -> (x-1=w75:i32)
            n223 = Equal?(x=w72, y=-1) -> ()  [unwired: 1 out]
            n224 = Build Array (concatenate)(w65, w69) -> (w70:dbl[][])
            n225 = for "Find nearest value to previous data set" {
              tunnel: w69 -> [w119] mode=indexing
              tunnel: w65 -> [w122]
              tunnel: [w118] -> w78 mode=indexing
              tunnel: w75 -> [w117]
              # "Calcs diffrences"
              # "Takes last data set"
              n226 = Index Array(array=w122, index (row)=w117) -> (element=w120:dbl[])  [unwired: 1 in]
              n227 = Subtract(x=w119, y=w120) -> (x-y=w121:dbl[])
              n228 = Absolute Value(x=w121) -> (abs(x)=w118:dbl[])
            }
            n229 = Increment(x=w61) -> (x+1=→"ProgBar top":i32)
            n230 = call "Peak tracking sq.vi"("BF len"=w59, "EnH choice"=w66, "Error control"="Tracking error limit", "Trace"=w61, "Poly count"=3, "Int IN"=w68, "Scan"=w70) -> ("Int Out"=w63:sgl[], "Scan Out"=w62:sgl[])  [unwired: 3 in]
            n231 = Build Array (concatenate)(w65, w62) -> (w64:dbl[][])
            n232 = Array Size(array=w69) -> (size(s)=w74:i32)
            n233 = for {
              N: w74 -> [_]
              shift-right: [w107] -> _
              shift-left: w78 -> [w105]
              shift-right: [w98] -> _
              shift-left: w74 -> [w99]
              tunnel: [w97] -> _ mode=indexing
              i -> [w108]
              # "Checks it's the smallest of all peaks"
              # "Finds smallest"
              n234 = Index Array(array=w105, index (col)=w108) -> (element=w102:dbl[])  [unwired: 1 in]
              n235 = Array Max & Min(array=w102) -> (min value=w101:dbl, min index (indices)=w106:i32)  [unwired: 2 out]
              n236 = Index Array(array=w105, index (row)=w106) -> (element=w104:dbl[])  [unwired: 1 in]
              n237 = Array Max & Min(array=w104) -> (min value=w103:dbl)  [unwired: 3 out]
              n238 = Equal?(x=w103, y=w101) -> (x = y?=w100:bool)
              n239 = case shown="True" w100 {
                tunnel: [w111 w115] -> w107
                tunnel: w106 -> [_ w114]
                tunnel: w105 -> [w111 w113]
                tunnel: w99 -> [w109 w112]
                tunnel: [w110 w112] -> w98
                tunnel: [w109 w112] -> w97
                frame False {
                  n240 = Increment(x=w109) -> (x+1=w110:i32)
                }
                frame True {
                  n241 = Replace Array Subset(array=w113, new element=dbl[] [], index (row)=w114) -> (w115:dbl[][])  [unwired: 1 in]
                }
              }
            }
          }
          n242 = Index Array(array=w40, index=0) -> (element=w38:i32)
          n243 = property on="ProgBar top" class="Slide (strict)"("Scale.Maximum"=w38) -> ()  [unwired: 2 in, 2 out]
          n244 = Transpose 2D Array(2D array=w35) -> (transposed array=w34:sgl[][])
          n245 = Transpose 2D Array(2D array=w33) -> (transposed array=w32:sgl[][])
          n246 = for {
            tunnel: w34 -> [w56] mode=indexing
            tunnel: w32 -> [w55] mode=indexing
            tunnel: [w56] -> w37 mode=indexing if=w53
            tunnel: [w55] -> w36 mode=indexing if=w53
            n247 = call "Crop Zero.vi"("Search data"=w56) -> ("Searched data out"=w58:dbl[])  [unwired: 3 in, 1 out]
            n248 = Array Size(array=w58) -> (size(s)=w54:i32)
            n249 = Greater?(x=w54, y="Minimum feature length") -> (0:w53:bool)
          }
          n250 = in-place-dvr #5(w29) -> (w27:errorcluster)  [unwired: 1 out]
        }
        "Feature positions" <- w25
        "Feature ampltuides" <- w24
        n251 = call <vilib>:"Clear Errors.vi"("error in (no error)"=w27) -> ()  [unwired: 5 in, 2 out]
      }
    }
    n252 = event shown="[1] \"Decimate Y/N\", \"Decimate\": Value Change" {
      selector: _ -> [_ _]
      dyn-events: _ -> [_ _]
      timeout: 10 -> [_ _]
      event Timeout {
        n253 = event-data() -> ()  [unwired: 1 in, 3 out]
      }
      event "Decimate Y/N", "Decimate": Value Change {
        # "Probably change this for something more efficent"
        n254 = event-data() -> ()  [unwired: 1 in, 6 out]
      }
    }
    n255 = disable-structure shown="Disabled" {
      frame Disabled {
        n256 = case shown="True" "Open feature settings" {
          frame False {
          }
          frame True {
            n257 = call "File Dialog"() -> ("selected path"=w16:path, "exists"=w15:bool, "error out"=w14:errorcluster)  [unwired: 12 in, 1 out]
            n258 = call <vilib>:"Clear Errors.vi"("error in (no error)"=w14) -> ()  [unwired: 5 in, 2 out]
            n259 = case shown="True" w15 {
              tunnel: w16 -> [_ w23]
              frame False {
              }
              frame True {
                n260 = call-poly <vilib>:"Read From Spreadsheet File.vi"("file path (dialog if empty)"=w23) -> ("all rows"=w22:string[][])  [unwired: 6 in, 4 out]
                n261 = Array Subset(array=w22, index (row)=0, length (row)=5) -> (w19:string[][])  [unwired: 2 in]
                n262 = Index Array(array=w19, index (col)=1) -> (element=w17:string[])  [unwired: 1 in]
                n263 = Index Array(array=w17) -> ()  [unwired: 5 in, 5 out]
                n264 = local read "Detection method"() -> ()  [unwired: 1 in]
                n265 = local read "Upper\nThreashold"() -> ()  [unwired: 1 in]
                n266 = local read "Lower\nThreashold"() -> ()  [unwired: 1 in]
                n267 = local read "Width"() -> ()  [unwired: 1 in]
                n268 = local read "2nd Derivative limit"() -> ()  [unwired: 1 in]
              }
            }
          }
        }
      }
      frame Enabled {
      }
    }
    n269 = case "Gets file name" shown="0, Default" "File style" {
      tunnel: [TRUE FALSE] -> w9
      frame 0, Default {
        n270 = local read "File displayed"() -> (w504:i32)
        n271 = local read "Files"() -> (w507:path[])
        n272 = Index Array(array=w507, index=w504) -> (element=w506:path)
        n273 = Strip Path(path=w506) -> (name=→"File\nname":string)  [unwired: 1 out]
      }
      frame 1 {
      }
    }
    n274 = case "Load up files list" shown="True" "Load files" {
      frame False {
      }
      frame True {
        n275 = local read "File style"() -> (w519:u16)
        n276 = local read "Files"() -> (w516:path[])
        n277 = local read "Xcol"() -> (w518:i16)
        n278 = local read "Ycol"() -> (w517:i16)
        n279 = call "Load data.vi"("File style in"=w519, "Fixed style"=FALSE, "Xcol in"=w518, "Ycol in"=w517, "Files in"=w516, "Delim in"="Delim") -> ("File style out"=w522:u16, "Xcol out"=w521:i16, "Ycol out"=w520:i16, "Files out"=w515:path[], "Delim out"=w514:string)  [unwired: 5 in]
        n280 = Array Size(array=w515) -> (size(s)=w511:i32)
        n281 = local write "File style"(w522) -> ()
        n282 = local write "Xcol"(w521) -> ()
        n283 = local write "Ycol"(w520) -> ()
        n284 = local write "Files"(w515) -> ()
        n285 = local write "Delim"(w514) -> ()
        n286 = Not Equal To 0?(x=w511) -> (x != 0?=w510:bool)
        n287 = local write "Load data"(w510) -> ()
      }
    }
    n288 = property on="File\nname" class="Str"("Visible"=w9) -> ()  [unwired: 2 in, 2 out]
    n289 = property on="Feature\ntype" class="CmbBox"() -> ("Value"=w3:string)  [unwired: 2 in, 2 out]
    n290 = Decimal String To Number(string=w3) -> (number=→"peaks/valleys":i32)  [unwired: 2 in, 1 out]
    n291 = case "Load zero data" shown="True" "Load zero" {
      frame False {
      }
      frame True {
        w210 = 0 ("File number to display")
        n292 = local read "Delim"() -> (w214:string)
        n293 = local read "Xcol"() -> (w216:i16)
        n294 = local read "Ycol"() -> (w215:i16)
        n295 = call "Load data.vi"("File style in"=0 ("File number to display"), "Fixed style"=TRUE, "Xcol in"=w216, "Ycol in"=w215, "Delim in"=w214) -> ("Xcol out"=w221:i16, "Ycol out"=w220:i16, "Files out"=w218:path[], "Delim out"=w219:string)  [unwired: 6 in, 1 out]
        n296 = call "File loader.vi"("File style in"=w210, "Files in"=w218, "File number to display"=w210, "Xcol"=w221, "Ycol"=w220, "Delim"=w219) -> ("Xdata"=→"Zero Xdata":dbl[], "Ydata"=→"Zero Ydata":dbl[])  [unwired: 11 in, 1 out]
      }
    }
    n297 = case shown="\"1st Scan\"" "Normalise\nmethod" {
      frame "All scans", Default {
      }
      frame "1st Scan" {
      }
    }
    n298 = case shown="True" "Load data" {
      frame False {
      }
      frame True {
        n299 = local read "teh data"() -> (w162:refnum<data-value>)
        n300 = in-place {
          n301 = in-place-match #6(w162) -> (w169:refnum<data-value>)
          n302 = local read "Files"() -> (w167:path[])
          n303 = Delete Data Value Reference(data value reference=w169) -> (error out=w168:errorcluster)  [unwired: 1 in, 1 out]
          n304 = call <vilib>:"Clear Errors.vi"("error in (no error)"=w168) -> ()  [unwired: 5 in, 2 out]
          n305 = local write "Load data"(FALSE) -> ()
          n306 = local read "File style"() -> (w166:u16)
          n307 = local read "Delim"() -> (w173:string)
          n308 = local read "Xcol"() -> (w175:i16)
          n309 = local read "Ycol"() -> (w174:i16)
          n310 = case shown="1" w166 {
            tunnel: [w184 w197] -> w177
            tunnel: w175 -> [w183 _]
            tunnel: w174 -> [w182 _]
            tunnel: w173 -> [w181 w202]
            tunnel: [w180 w196] -> w172
            tunnel: w167 -> [w179 w205]
            tunnel: [w178 w194] -> w165
            frame 0, Default {
              n311 = Array Size(array=w179) -> (size(s)=w178:i32)
              n312 = for {
                N: w178 -> [_]
                tunnel: w179 -> [w191]
                tunnel: [w192] -> w184
                tunnel: [w193] -> w180 mode=indexing
                tunnel: w183 -> [w190]
                tunnel: w182 -> [w189]
                tunnel: w181 -> [w188]
                i -> [w187]
                n313 = Index Array(array=w191, index=w187) -> (element=w185:path)
                n314 = call-poly <vilib>:"Read From Spreadsheet File.vi"("delimiter (\\t)"=w188, "file path (dialog if empty)"=w185) -> ("all rows"=w186:dbl[][])  [unwired: 5 in, 4 out]
                n315 = Index Array(array=w186, index (col) #1=w190, index (col) #2=w189) -> (element #1=w192:dbl[], element #2=w193:dbl[])  [unwired: 2 in]
              }
            }
            frame 1 {
              n316 = Index Array(array=w205, index=0) -> (element=w203:path)
              n317 = call-poly <vilib>:"Read From Spreadsheet File.vi"("delimiter (\\t)"=w202, "file path (dialog if empty)"=w203) -> ("all rows"=w199:dbl[][])  [unwired: 5 in, 4 out]
              n318 = Array Size(array=w199) -> (size(s)=w201:i32[])
              n319 = Index Array(array=w199, index (col)=0) -> (element=w197:dbl[])  [unwired: 1 in]
              n320 = Index Array(array=w201, index=1) -> (element=w195:i32)
              n321 = Decrement(x=w195) -> (x-1=w194:i32)
              n322 = for {
                N: w194 -> [_]
                tunnel: w199 -> [w209]
                tunnel: [w208] -> w196 mode=indexing
                i -> [w207]
                n323 = Increment(x=w207) -> (x+1=w206:i32)
                n324 = Index Array(array=w209, index (col)=w206) -> (element=w208:dbl[])  [unwired: 1 in]
              }
            }
          }
          "Wavelengths" <- w177
          "Number of files" <- w165
          n325 = Transpose 2D Array(2D array=w172) -> (transposed array=w171:dbl[][])
          n326 = Decrement(x=w165) -> (x-1=w164:i32)
          n327 = New Data Value Reference(data value=w171) -> (data value reference=w170:refnum<data-value>)  [unwired: 1 in, 1 out]
          n328 = property on="File displayed" class="Slide (strict)"("Maximum"=w164, "Scale.Maximum"=w164) -> ()  [unwired: 2 in, 2 out]
          n329 = in-place-match #6(w170) -> (→"teh data":refnum<data-value>)
        }
      }
    }
  }
